vi "UpdateSensorReadings.vi"(10 "Data in":dbl, 11 "Cluster in":cluster{"SensorCluster":T1}) -> (3 "Cluster out":cluster{"SensorCluster":T1})   [LabVIEW 2018]
uses:
  Type_Def/Type_Def ClusterSensor.ctl
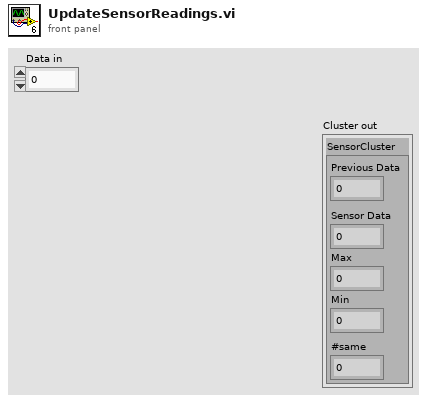
[diagram p1: front panel]
types:
  T1 = typedef "Type_Def ClusterSensor.ctl" = cluster{"Sensor Data":dbl, "Max":dbl, "Min":dbl, "Previous Data":dbl, "#same":dbl}
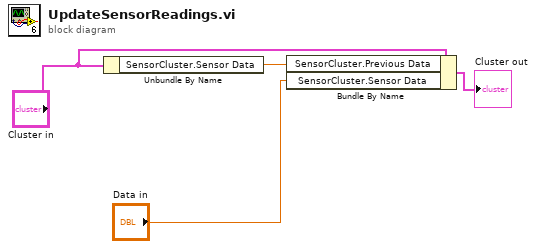
[diagram p0: block diagram]
diagram:
  n1 = Unbundle By Name("Cluster in") -> ("SensorCluster.Sensor Data"=w2:dbl)
  n2 = Bundle By Name(cluster="Cluster in", "SensorCluster.Previous Data"=w2, "SensorCluster.Sensor Data"="Data in") -> (→"Cluster out":cluster{"SensorCluster":T1})
